vi "Init.vi"(8 "error in (no error)":errorcluster, 10 "Index":i32, 11 "Group":refnum<class "Group STR.lvclass">) -> (0 "error out":errorcluster, 3 "StringChannel out":refnum<class "Channel STR.lvclass">)   [LabVIEW 2020, in "Vecto.lvlib" / "Channel STR.lvclass"]
uses:
  Channel STR.lvclass
  Group STR/Group STR.lvclass
  Channel STR.lvclass/Channel STR.ctl
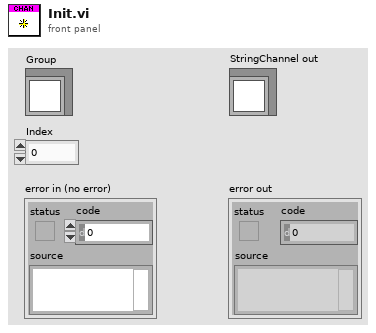
[diagram p1: front panel]
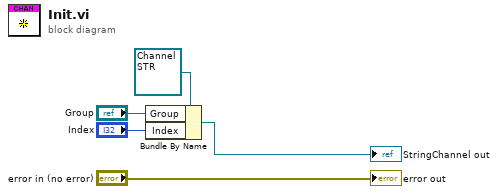
[diagram p0: block diagram]
diagram:
  n1 = Bundle By Name(cluster=refnum<class "Channel STR.lvclass"> refnum ("StringChannel in"), "Group"="Group", "Index"="Index") -> (→"StringChannel out":refnum<class "Channel STR.lvclass">)
  "error out" <- "error in (no error)"
